vi "Write wrapnum.vi"(8 "error in (no error)":errorcluster, 10 "wrapnum":T1, 11 "Wrapnum.lvclass in":refnum<class "Wrapnum.lvclass">) -> (0 "error out":errorcluster, 3 "Wrapnum.lvclass out":refnum<class "Wrapnum.lvclass">)   [LabVIEW 2010, in "TCS.lvlib" / "TCSDataDefinitions.lvlib" / "TCSCommand.lvlib" / "Wrapnum.lvclass"]
uses:
  Wrapnum.lvclass
  Enumerations/WrapnumTypes.ctl
  Wrapnum.lvclass/Wrapnum.ctl
  TCSCommand.lvlib
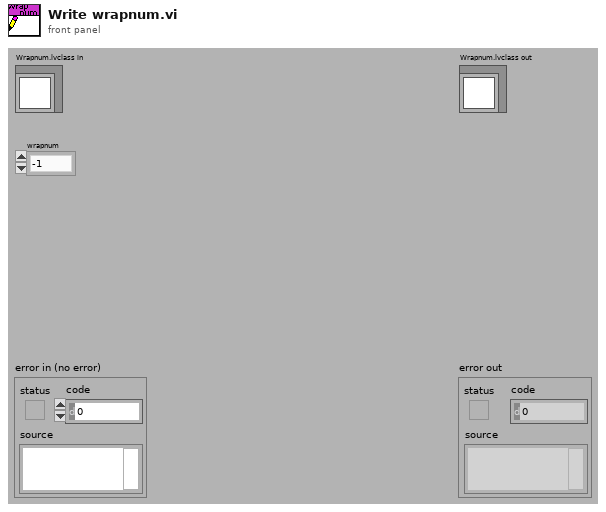
[diagram p1: front panel]
types:
  T1 = typedef "TCS.lvlib/TCSDataDefinitions.lvlib/TCSCommand.lvlib/WrapnumTypes.ctl" = enum16{"-1", "0", "1"}
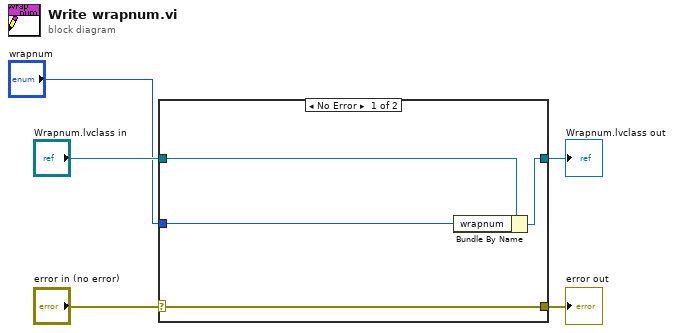
[diagram p0: block diagram]
diagram:
  n1 = case shown="No Error" "error in (no error)" {
    selector: "error in (no error)" -> [w9 w10]
    tunnel: [w9 w10] -> w4
    tunnel: [w7 w11] -> w2
    tunnel: "Wrapnum.lvclass in" -> [w8 w11]
    tunnel: "wrapnum" -> [w6 _]
    frame No Error {
      n2 = Bundle By Name(cluster=w8, "wrapnum"=w6) -> (w7:refnum<class "Wrapnum.lvclass">)
    }
    frame Error {
    }
  }
  "error out" <- w4
  "Wrapnum.lvclass out" <- w2
